vi "Get Module Main VI Information.vi"(8 "error in (no error)":errorcluster) -> (0 "error out":errorcluster, 1 "Execution State":T1(ring), 2 "Is Module Running?":bool, 3 "Module Main VI":refnum<vi>)   [LabVIEW 2022 SP3, in "Event Manager.lvlib"]
doc: "Return information about the module main VI, including its VI reference, its execution state enum, and a Boolean value indicating whether or not it is running.\n____\nHAMPEL SOFTWARE ENGINEERING v2.6.0 (2023-12-19 10:54)"
uses:
  Event Manager.lvlib
  Main.vi
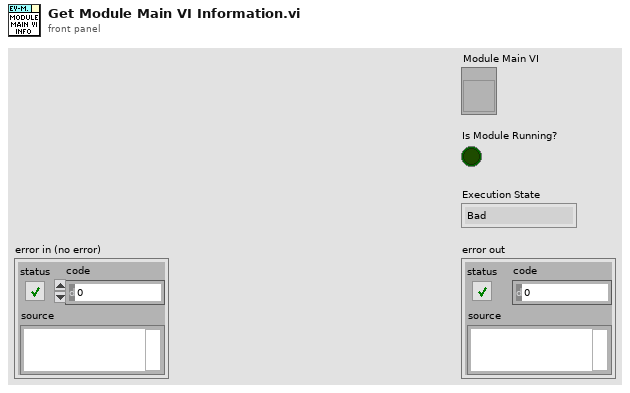
[diagram p1: front panel]
types:
  T1 = enum32{"Bad", "Idle", "Run top level", "Running"}
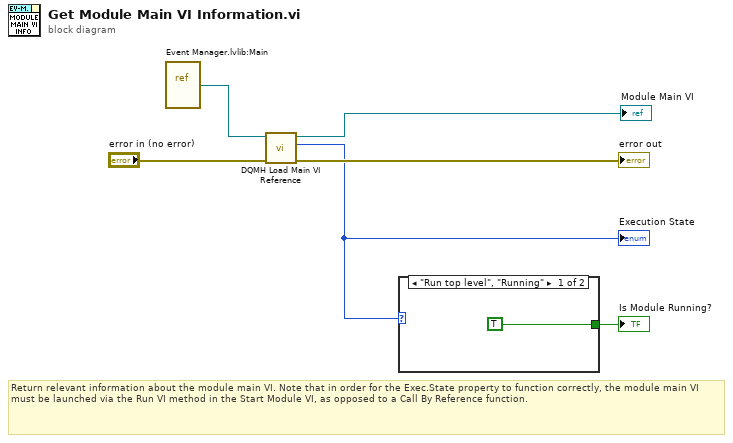
[diagram p0: block diagram]
diagram:
  # "Return relevant information about the module main VI. Note that in order for the Exec.State property to function correctly, the module main VI must be launched via the Run VI method in the Start Module VI, as opposed to a Call By Reference function."
  n1 = vi-ref "Event Manager.lvlib:Main.vi"() -> (w2:refnum<vi>)
  n2 = call "DQMH Load Main VI Reference.vi"("error in (no error)"="error in (no error)", "VI in"=w2) -> ("error out"=→"error out":errorcluster, "Execution:State"=w3:T1, "VI out"=→"Module Main VI":refnum<vi>)  [unwired: 7 in]
  "Execution State" <- w3
  n3 = case shown="\"Run top level\", \"Running\"" w3 {
    tunnel: [TRUE _] -> w6
    frame "Run top level", "Running" {
    }
    frame "Bad", "Idle" {
    }
  }
  "Is Module Running?" <- w6
